vi "Error Query.vi"(8 "error in (no error)":errorcluster, 11 "VISA resource name":refnum<visa-resource-name>) -> (0 "error out":errorcluster, 1 "Error Message":string, 2 "Error Code":i32[](array[numeric]), 3 "VISA resource name out":refnum<visa-resource-name>)   [LabVIEW 2012, in "Tektronix DPO MSO 2000 4000 Series.lvlib"]
doc: "Queries an instrument for any errors in the error queue of the instrument. The Error Query VI continuously reads errors until this VI reads all the errors from the instrument. \n<B>Note</B>: Because most driver VIs automatically call the Error Query VI, you do not need to call this VI in an application."
uses:
  <instrlib>/Tektronix DPO MSO 2000 4000 Series/Tektronix DPO MSO 2000 4000 Series.lvlib
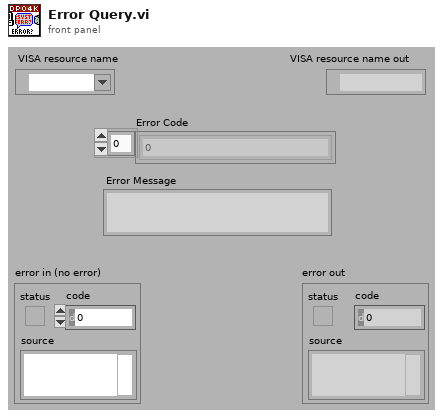
[diagram p1: front panel]
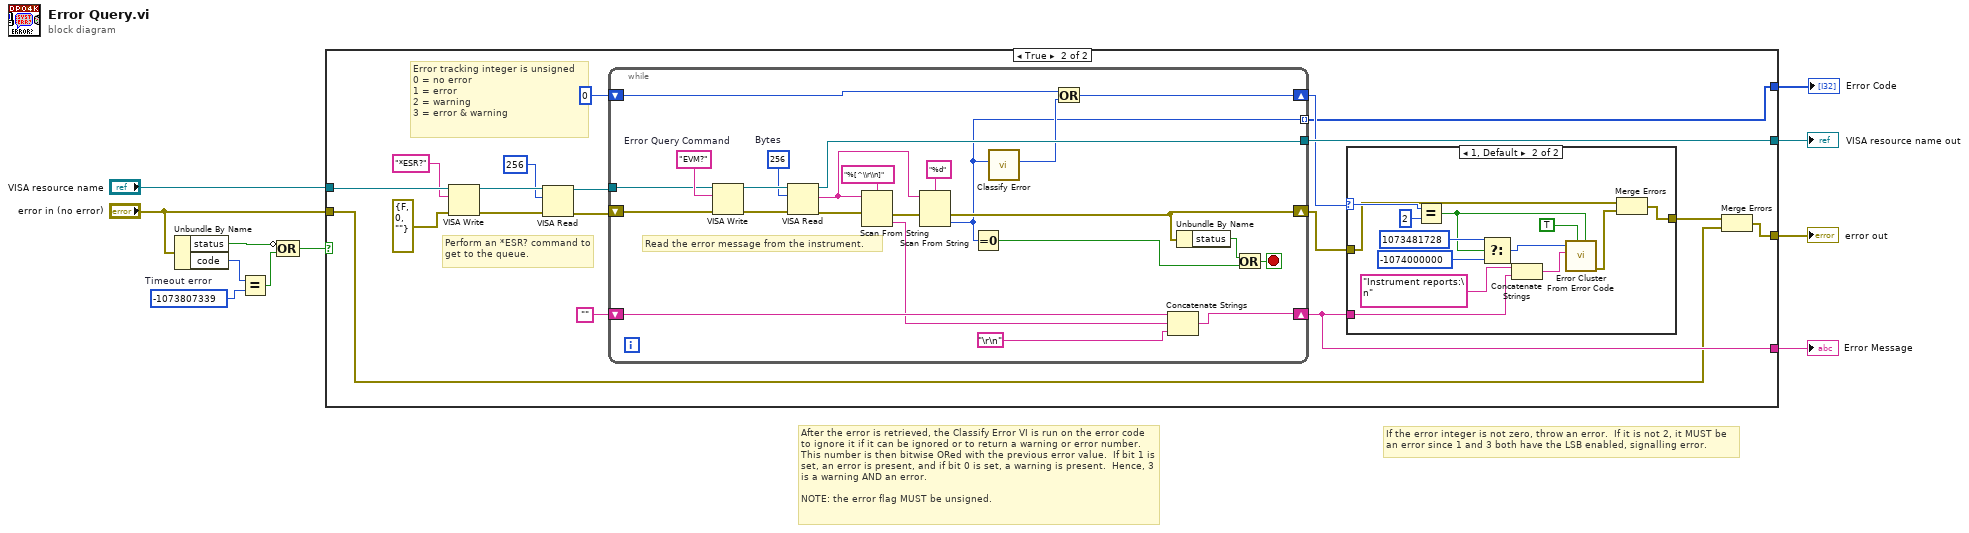
[diagram p0: block diagram]
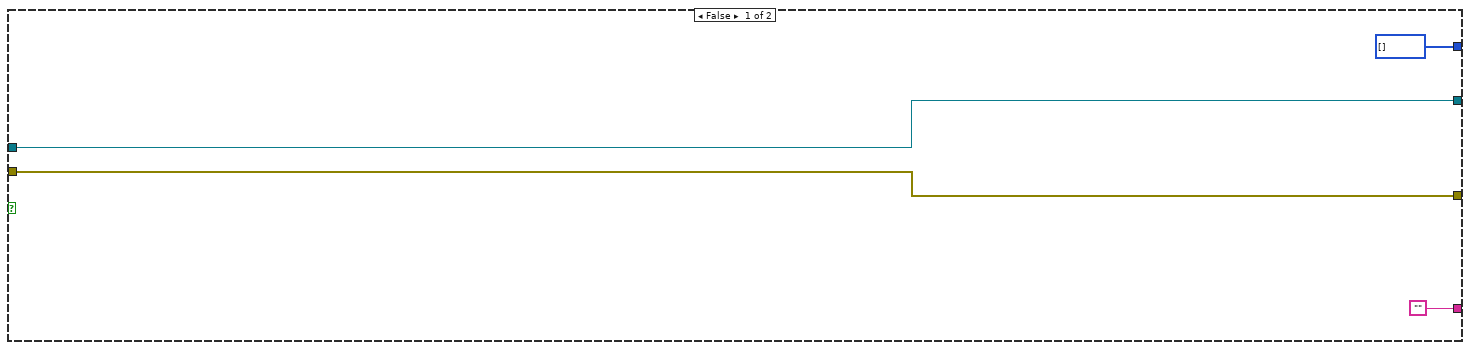
[diagram p2: hidden frame]
diagram:
  w6 = -1073807339  # Timeout error
  # "If the error integer is not zero, throw an error.  If it is not 2, it MUST be an error since 1 and 3 both have the LSB enabled, signalling error."
  # "After the error is retrieved, the Classify Error VI is run on the error code to ignore it if it can be ignored or to return a warning or error number.  This number is then bitwise ORed with the previous error value.  If bit 1 is set, an error is present, and if bit 0 is set, a warning is present.  Hence, 3 is a warning AND an error.\n\nNOTE: the error flag MUST be unsigned."
  n1 = Unbundle By Name("error in (no error)") -> ("status"=w7:bool, "code"=w4:i32)
  n2 = Equal?(x=w4, y=w6) -> (x = y?=w5:bool)
  n3 = Compound Arithmetic op=OR(invert w7, w5) -> (w3:bool)
  n4 = case shown="True" w3 {
    tunnel: [w15 w33] -> w11
    tunnel: "VISA resource name" -> [w15 w29]
    tunnel: "error in (no error)" -> [w14 w16]
    tunnel: [w14 w31] -> w9
    tunnel: ["" w30] -> w2
    tunnel: [i32[] [] w18] -> w1
    frame False {
    }
    frame True {
      # "Error tracking integer is unsigned\n0 = no error\n1 = error\n2 = warning\n3 = error & warning"
      # "Perform an *ESR? command to get to the queue."
      n5 = VISA Write(VISA resource name=w29, write buffer="*ESR?", error in (no error)=errorcluster {"status"=FALSE, "code"=0, "source"=""}) -> (VISA resource name out=w26:refnum<visa-resource-name>, error out=w27:errorcluster)  [unwired: 1 out]
      n6 = VISA Read(VISA resource name=w26, byte count=u32 256, error in (no error)=w27) -> (VISA resource name out=w24:refnum<visa-resource-name>, error out=w23:errorcluster)  [unwired: 2 out]
      n7 = while {
        tunnel: [w71] -> w33
        tunnel: w24 -> [w54]
        shift-right: [w60] -> w30
        shift-left: "" -> [w62]
        shift-right: [w51] -> w21
        shift-left: u32 0 ("x = 0?") -> [w50]
        shift-right: [w58] -> w20
        shift-left: w23 -> [w59]
        tunnel: [w48] -> w18 mode=indexing
        stop <- w65 stop-if-true
        w69 = u32 256  # Bytes
        w67 = "EVM?"  # Error Query Command
        # "Read the error message from the instrument."
        n8 = VISA Write(VISA resource name=w54, write buffer=w67, error in (no error)=w59) -> (VISA resource name out=w70:refnum<visa-resource-name>, error out=w68:errorcluster)  [unwired: 1 out]
        n9 = VISA Read(VISA resource name=w70, byte count=w69, error in (no error)=w68) -> (VISA resource name out=w71:refnum<visa-resource-name>, read buffer=w63:string, error out=w57:errorcluster)  [unwired: 1 out]
        n10 = Scan From String(format string="%[^\\r\\n]", input string=w63, error in=w57) -> (error out=w56:errorcluster, output 1=w61:string)  [unwired: 2 in, 2 out]
        n11 = Scan From String(format string="%d", input string=w63, error in=w56) -> (error out=w58:errorcluster, output 1=w48:i32)  [unwired: 2 in, 2 out]
        n12 = Equal To 0?(x=w48) -> (x = 0?=w53:bool)
        n13 = call <instrlib>:"Classify Error.vi"("Error Code"=w48) -> ("Error Classification"=w49:i32)  [unwired: 10 in]
        n14 = Or(x=w50, y=w49) -> (x .or. y?=w51:u32)
        n15 = Concatenate Strings(w62, w61, "\r\n") -> (w60:string)
        n16 = Unbundle By Name(w58) -> ("status"=w55:bool)
        n17 = Or(x=w55, y=w53) -> (x .or. y?=w65:bool)
      }
      n18 = case shown="1, Default" w21 {
        selector: w21 -> [_ w43]
        tunnel: [w34 w35] -> w17
        tunnel: w30 -> [_ w44]
        tunnel: w20 -> [w34 w37]
        frame 0 {
        }
        frame 1, Default {
          n19 = Equal?(x=w43, y=u32 2) -> (x = y?=w40:bool)
          n20 = Select(t=1073481728 ("Code"), s=w40, f=-1074000000 ("Code")) -> (s? t:f=w38:i32)
          n21 = Concatenate Strings("Instrument reports:\n" ("Source"), w44) -> (w45:string)
          n22 = call <vilib>:"Error Cluster From Error Code.vi"("is warning? (False)"=w40, "show call chain? (False)"=TRUE, "error message (\"\")"=w45, "error code (0)"=w38) -> ("error out"=w36:errorcluster)  [unwired: 5 in]
          n23 = Merge Errors(w37, w36) -> (w35:errorcluster)
        }
      }
      n24 = Merge Errors(w17, w16) -> (w31:errorcluster)
    }
  }
  "VISA resource name out" <- w11
  "error out" <- w9
  "Error Message" <- w2
  "Error Code" <- w1
